vi "restart.vi"   [LabVIEW 2015]
uses:
  <vilib>/nisyscfg/nisyscfg.lvlib
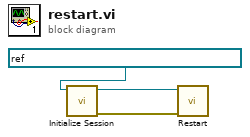
[diagram p0: block diagram]
diagram:
  n1 = call <vilib>:"Initialize Session.vi"("Target (localhost)"=refnum<k21> "NI-PXIe8135-2F217AF0 (192.168.150.78)" ("Session in")) -> ("error out"=w2:errorcluster, "Session out"=w3:refnum<k21>)  [unwired: 9 in]
  n2 = call <vilib>:"Restart.vi"("error in (no error)"=w2, "Session in"=w3) -> ()  [unwired: 7 in, 3 out]
